vi "ARI Control.vi"(4 "ARI Input Controls":T1) -> (1 "ARI Output Controls":T1)   [LabVIEW 2015]
uses:
  <vilib>/Rock Robotics/WPI/Relay/WPI_RelayValue.ctl
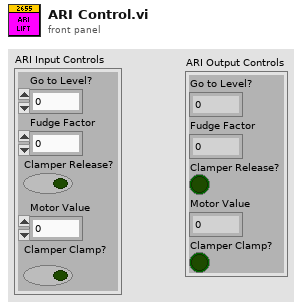
[diagram p1: front panel]
types:
  T1 = cluster{"Go to Level?":i32, "Fudge Factor":dbl, "Clamper Release?":bool, "Motor Value":dbl, "Clamper Clamp?":bool}
  T2 = typedef "WPI_SwitchDevRef.ctl" = cluster{"DevStatus":errorcluster, "DIO Channel":T3, "CntIndex":T4, "Normally Closed":bool}
  T3 = typedef "FPGA_DIOChannel.ctl" = enum8{"DIO 0", "DIO 1", "DIO 2", "DIO 3", "DIO 4", "DIO 5", "DIO 6", "DIO 7", "DIO 8", "DIO 9", "DIO MXP 0", "DIO MXP 1", "DIO MXP 2", "DIO MXP 3", "DIO MXP 4", "DIO MXP 5", "DIO MXP 6", "DIO MXP 7", "DIO MXP 8", "DIO MXP 9", "DIO MXP 10", "DIO MXP 11", "DIO MXP 12", "DIO MXP 13", "DIO MXP 14", "DIO MXP 15", "Invalid"}
  T4 = typedef "FPGA_CounterCtrSystemIndex.ctl" = enum8{"Ctr 0", "Ctr 1", "Ctr 2", "Ctr 3", "Ctr 4", "Ctr 5", "Ctr 6", "Ctr 7", "Invalid"}
  T5 = typedef "WPI_RelayValue.ctl" = enum16{"Off", "On", "Forward", "Reverse"}
  T6 = typedef "WPI_RelayDevRef.ctl" = cluster{"DevStatus":errorcluster, "Relay Channel":T7, "Relay Direction":T8}
  T7 = typedef "FPGA_DIORelayChannel.ctl" = enum8{"Relay 0", "Relay 1", "Relay 2", "Relay 3", "Invalid"}
  T8 = typedef "WPI_RelayDirection.ctl" = enum16{"Both directions", "Forward only", "Reverse only"}
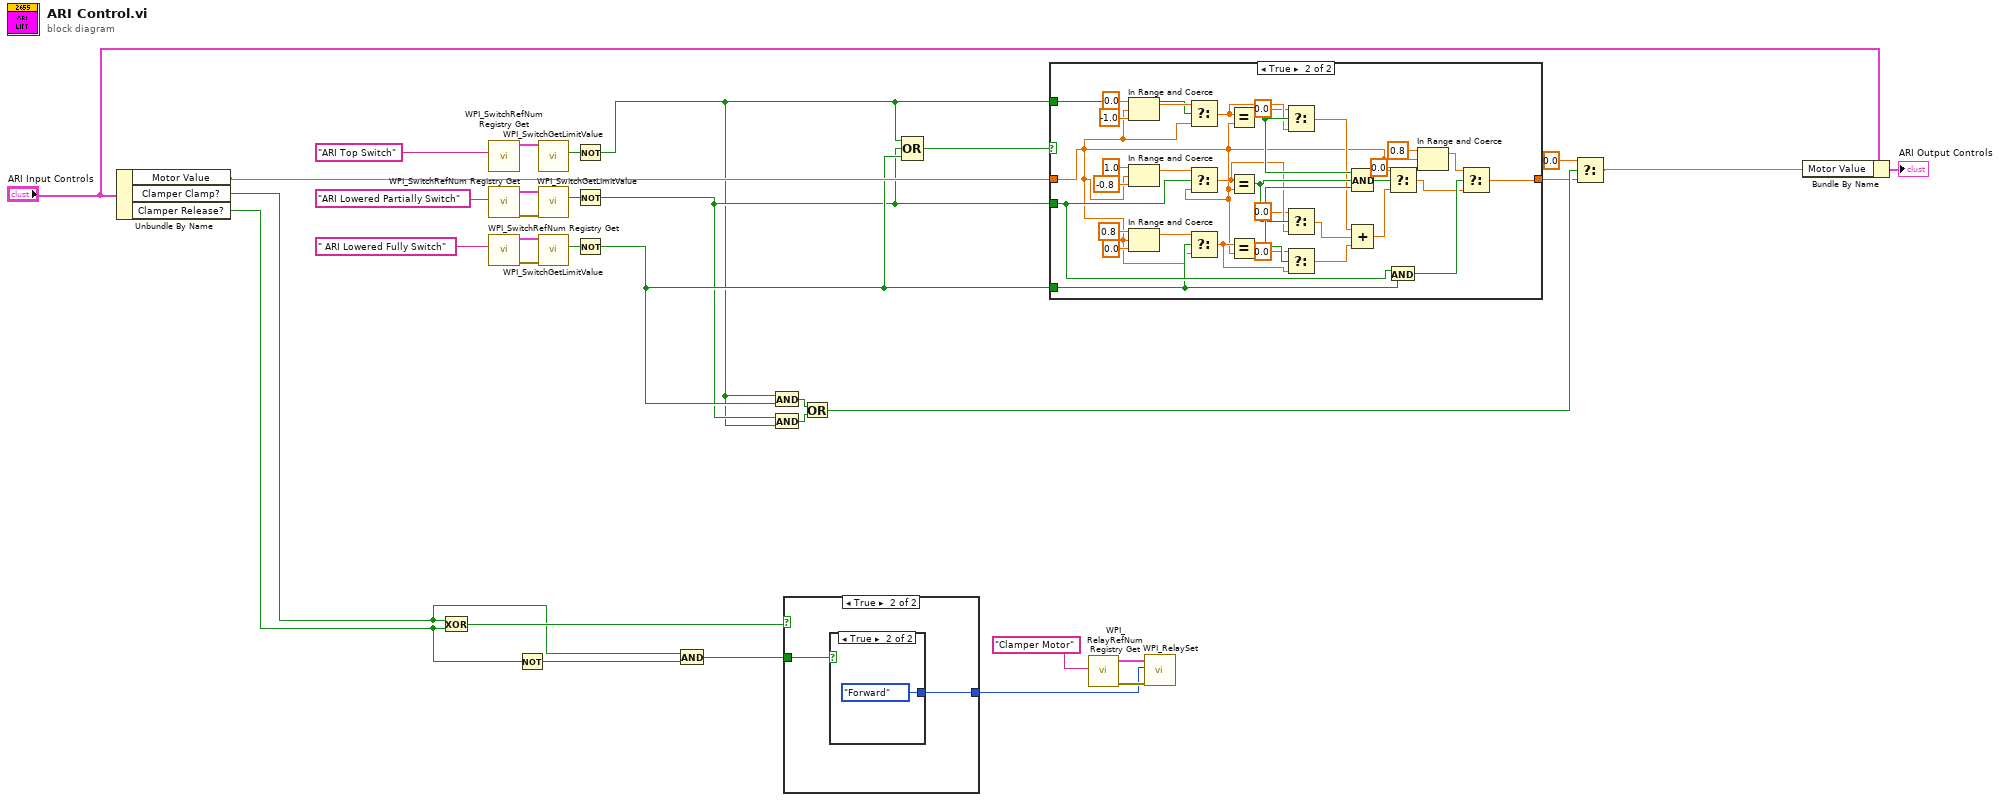
[diagram p0: block diagram]
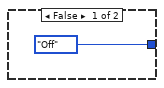
[diagram p3: hidden frame]
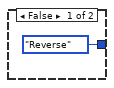
[diagram p4: hidden frame]
diagram:
  n1 = Unbundle By Name("ARI Input Controls") -> ("Motor Value"=w10:dbl, "Clamper Clamp?"=w20:bool, "Clamper Release?"=w22:bool)
  n2 = Exclusive Or(1:w22, 2:w20) -> (0:w24:bool)
  n3 = call <vilib>:"WPI_SwitchRefNum Registry Get.vi"("refnum name"="ARI Top Switch") -> ("SwitchDevRef"=w18:T2)  [unwired: 9 in, 1 out]
  n4 = call <vilib>:"WPI_SwitchRefNum Registry Get.vi"("refnum name"="ARI Lowered Partially Switch") -> ("error out"=w31:errorcluster, "SwitchDevRef"=w32:T2)  [unwired: 9 in]
  n5 = call <vilib>:"WPI_SwitchRefNum Registry Get.vi"("refnum name"=" ARI Lowered Fully Switch") -> ("error out"=w29:errorcluster, "SwitchDevRef"=w28:T2)  [unwired: 9 in]
  n6 = Not(x=w22) -> (.not. x?=w21:bool)
  n7 = call <vilib>:"WPI_SwitchGetLimitValue.vi"("SwitchDevRef"=w18) -> ("Switch Pressed"=w9:bool)  [unwired: 8 in, 2 out]
  n8 = call <vilib>:"WPI_SwitchGetLimitValue.vi"("error in (no error)"=w31, "SwitchDevRef"=w32) -> ("Switch Pressed"=w8:bool)  [unwired: 7 in, 2 out]
  n9 = call <vilib>:"WPI_SwitchGetLimitValue.vi"("error in (no error)"=w29, "SwitchDevRef"=w28) -> ("Switch Pressed"=w7:bool)  [unwired: 7 in, 2 out]
  n10 = Not(x=w9) -> (.not. x?=w1:bool)
  n11 = Not(x=w8) -> (.not. x?=w2:bool)
  n12 = Not(x=w7) -> (.not. x?=w3:bool)
  n13 = And(x=w20, y=w21) -> (x .and. y?=w19:bool)
  n14 = And(x=w1, y=w3) -> (x .and. y?=w15:bool)
  n15 = And(x=w2, y=w1) -> (x .and. y?=w14:bool)
  n16 = case shown="True" w24 {
    tunnel: [WPI_RelayValue."Off" ("RelayValue") w35] -> w23
    tunnel: w19 -> [_ w36]
    frame False {
    }
    frame True {
      n17 = case shown="True" w36 {
        tunnel: [WPI_RelayValue."Reverse" ("RelayValue") WPI_RelayValue."Forward" ("RelayValue")] -> w35
        frame False {
        }
        frame True {
        }
      }
    }
  }
  n18 = Or(x=w15, y=w14) -> (x .or. y?=w13:bool)
  n19 = Compound Arithmetic op=OR(w1, w2, w3) -> (w12:bool)
  n20 = case shown="True" w12 {
    tunnel: w3 -> [_ w47]
    tunnel: w2 -> [_ w48]
    tunnel: w10 -> [w39 w42]
    tunnel: w1 -> [_ w63]
    tunnel: [w39 w44] -> w11
    frame False {
    }
    frame True {
      n21 = In Range and Coerce(upper limit=0.0, x=w42, lower limit=-1.0) -> (coerced(x)=w66:dbl)  [unwired: 1 out]
      n22 = In Range and Coerce(upper limit=1.0, x=w42, lower limit=-0.8) -> (coerced(x)=w69:dbl)  [unwired: 1 out]
      n23 = In Range and Coerce(upper limit=0.8, x=w42, lower limit=0.0) -> (coerced(x)=w72:dbl)  [unwired: 1 out]
      n24 = Select(t=w66, s=w63, f=w42) -> (s? t:f=w51:dbl)
      n25 = Select(t=w69, s=w48, f=w42) -> (s? t:f=w54:dbl)
      n26 = Select(t=w72, s=w47, f=w42) -> (s? t:f=w53:dbl)
      n27 = Equal?(x=w51, y=w42) -> (x = y?=w60:bool)
      n28 = Equal?(x=w54, y=w42) -> (x = y?=w61:bool)
      n29 = Equal?(x=w53, y=w42) -> (x = y?=w62:bool)
      n30 = Select(t=0.0, s=w60, f=w51) -> (s? t:f=w59:dbl)
      n31 = Select(t=0.0, s=w61, f=w54) -> (s? t:f=w57:dbl)
      n32 = Select(t=0.0, s=w62, f=w53) -> (s? t:f=w58:dbl)
      n33 = Compound Arithmetic op=AND(w60, w61, w62) -> (w56:bool)
      n34 = Compound Arithmetic op=ADD(w59, w57, w58) -> (w55:dbl)
      n35 = Select(t=w42, s=w56, f=w55) -> (s? t:f=w45:dbl)
      n36 = And(x=w48, y=w47) -> (x .and. y?=w46:bool)
      n37 = In Range and Coerce(upper limit=0.8, x=w42, lower limit=0.0) -> (coerced(x)=w43:dbl)  [unwired: 1 out]
      n38 = Select(t=w43, s=w46, f=w45) -> (s? t:f=w44:dbl)
    }
  }
  n39 = call <vilib>:"WPI_RelayRefNum Registry Get.vi"("refnum name"="Clamper Motor") -> ("error out"=w26:errorcluster, "RelayDevRef"=w25:T6)  [unwired: 9 in]
  n40 = call <vilib>:"WPI_RelaySet.vi"("error in (no error)"=w26, "RelayValue"=w23, "RelayDevRef"=w25) -> ()  [unwired: 7 in, 2 out]
  n41 = Select(t=0.0, s=w13, f=w11) -> (s? t:f=w6:dbl)
  n42 = Bundle By Name(cluster="ARI Input Controls", "Motor Value"=w6) -> (→"ARI Output Controls":T1)
